vi "Log_Path_Header.vi"(8 "error in":errorcluster, 10 "File Name":string, 11 "start path":path=path "D:/DataLog") -> (0 "error out":errorcluster, 3 "path":path)   [LabVIEW 2018]
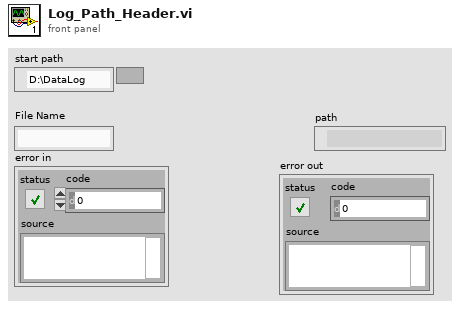
[diagram p1: front panel]
types:
  T1 = enum16{"open", "replace", "create", "open or create", "replace or create", "replace or create with confirmation"}
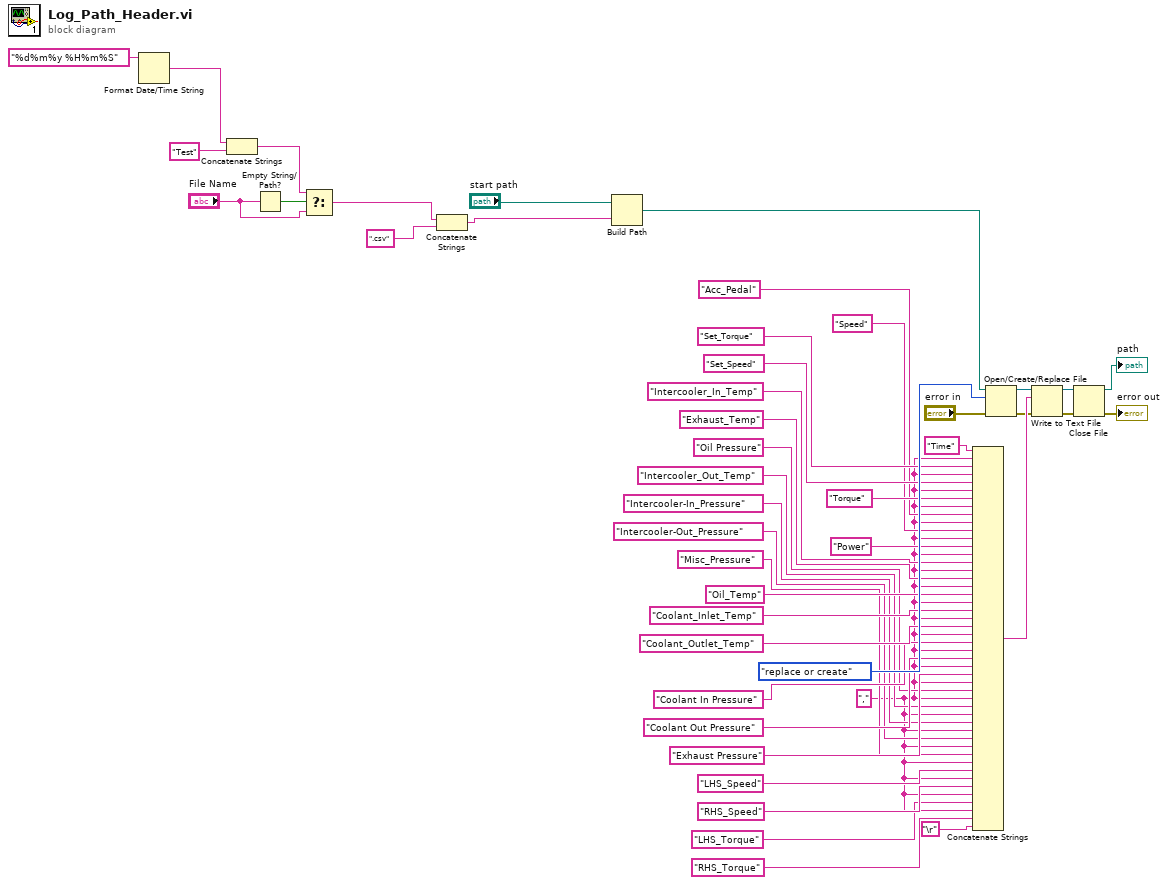
[diagram p0: block diagram]
diagram:
  w14 = ","
  n1 = Format Date/Time String(time format string (%c)="%d%m%y %H%m%S") -> (date/time string=w1:string)  [unwired: 2 in]
  n2 = Concatenate Strings(w1, "Test" ("string")) -> (w6:string)
  n3 = Empty String/Path?(string/path="File Name") -> (empty?=w7:bool)
  n4 = Select(t=w6, s=w7, f="File Name") -> (s? t:f=w3:string)
  n5 = Concatenate Strings(w3, ".csv" ("string")) -> (w9:string)
  n6 = Build Path(base path="start path", name or relative path=w9) -> (appended path=w11:path)
  n7 = Concatenate Strings("Time" ("string"), w14, "Set_Torque" ("string"), w14, "Set_Speed" ("string"), w14, "Torque" ("string"), w14, "Acc_Pedal" ("string"), w14, "Speed" ("string"), w14, "Power" ("string"), w14, "Intercooler_In_Temp" ("string"), w14, "Exhaust_Temp" ("string"), w14, "Oil_Temp" ("string"), w14, "Coolant_Inlet_Temp" ("string"), w14, "Coolant_Outlet_Temp" ("string"), w14, "Coolant In Pressure" ("string"), w14, "Coolant Out Pressure" ("string"), w14, "Exhaust Pressure" ("string"), w14, "Oil Pressure" ("string"), w14, "Intercooler_Out_Temp" ("string"), w14, "Intercooler-In_Pressure" ("string"), w14, "Intercooler-Out_Pressure" ("string"), w14, "Misc_Pressure" ("string"), w14, "LHS_Speed" ("string"), w14, "RHS_Speed" ("string"), w14, "LHS_Torque" ("string"), w14, "RHS_Torque" ("string"), "\r") -> (w46:string)
  n8 = Open/Create/Replace File(file path (use dialog)=w11, error in="error in", operation (0:open)=T1."replace or create") -> (refnum out=w42:refnum<file>, error out=w43:errorcluster)  [unwired: 3 in, 1 out]
  n9 = Write to Text File(file (use dialog)=w42, text=w46, error in=w43) -> (refnum out=w45:refnum<file>, error out=w44:errorcluster)  [unwired: 1 in, 1 out]
  n10 = Close File(refnum=w45, error in=w44) -> (path=→"path":path, error out=→"error out":errorcluster)
